vi "Get Line Filter.vi"(8 "error in (no error)":errorcluster, 11 "VISA resource name":refnum<visa-resource-name>) -> (0 "error out":errorcluster, 2 "Line Frequency Rejection":T1, 3 "VISA resource name out":refnum<visa-resource-name>)   [LabVIEW 2016, in "SR7270 Drivers.lvclass"]
uses:
  SR7270 Drivers.lvclass
  Typedefs/LF--enum.ctl
panel:
  out "f (0=60 Hz, 1=50 Hz)":string
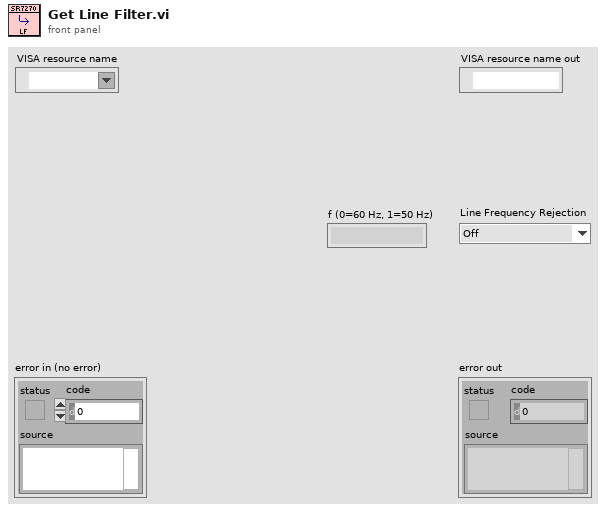
[diagram p1: front panel]
types:
  T1 = typedef "SR7270 Drivers.lvclass/LF--enum.ctl" = enum16{"Off", "60 Hz", "120 Hz", "60 & 120 Hz"}
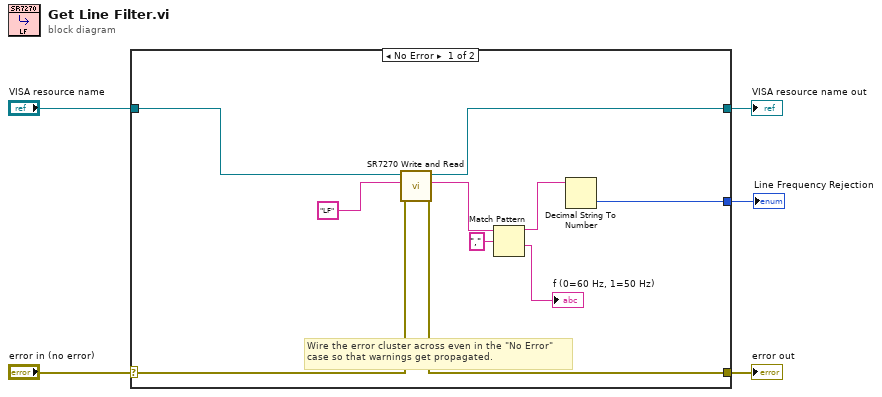
[diagram p0: block diagram]
diagram:
  n1 = case shown="No Error" "error in (no error)" {
    selector: "error in (no error)" -> [w15 w17]
    tunnel: [w14 w17] -> w4
    tunnel: [w6 w16] -> w2
    tunnel: "VISA resource name" -> [w7 w16]
    tunnel: [w12 _] -> w1
    frame No Error {
      # "Wire the error cluster across even in the \"No Error\"\ncase so that warnings get propagated."
      n2 = call "SR7270 Write and Read.vi"("error in (no error)"=w15, "Command Name"="LF", "VISA resource name"=w7) -> ("error out"=w14:errorcluster, "Read"=w11:string, "VISA resource name out"=w6:refnum<visa-resource-name>)  [unwired: 5 in, 1 out]
      n3 = Match Pattern(string=w11, regular expression=",") -> (before substring=w9:string, after substring=→"f (0=60 Hz, 1=50 Hz)":string)  [unwired: 1 in, 2 out]
      n4 = Decimal String To Number(string=w9) -> (number=w12:i32)  [unwired: 2 in, 1 out]
    }
    frame Error {
    }
  }
  "error out" <- w4
  "VISA resource name out" <- w2
  "Line Frequency Rejection" <- w1
